vi "GetTimeStamp.vi"(10 "ErrorIn":errorcluster) -> (2 "ErrorOut":errorcluster, 3 "TimeOut":dbl)   [LabVIEW 2018]
doc: "Returns the current time stamp, in seconds, elapsed since 12:00 a.m., Friday, January 1, 1904, Universal Time.\n\nError Clusters In and Out allow for this to be called with forced data flow.\n\nCopyright © 2019 Epimedia, Inc. All Rights Reserved.\n\nThe Epimedia Application Library is Copyright © 2009-2017 Epimedia, Inc. \nAll Rights Reserved. Used under license."
panel:
  # "Copyright © 2019 Epimedia, Inc. All Rights Reserved.\n\nThe Epimedia Application Library is Copyright © 2009-2017 Epimedia, Inc. \nAll Rights Reserved. Used under license."
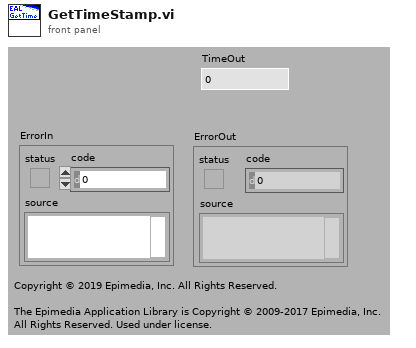
[diagram p1: front panel]
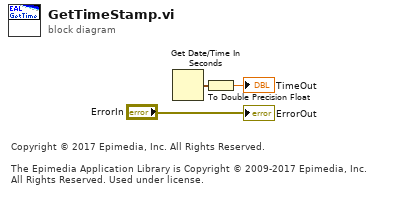
[diagram p0: block diagram]
diagram:
  # "Copyright © 2017 Epimedia, Inc. All Rights Reserved.\n\nThe Epimedia Application Library is Copyright © 2009-2017 Epimedia, Inc. \nAll Rights Reserved. Used under license."
  n1 = Get Date/Time In Seconds() -> (seconds since 1Jan1904=w2:timestamp)
  n2 = To Double Precision Float(number=w2) -> (double precision float=→"TimeOut":dbl)
  "ErrorOut" <- "ErrorIn"
